vi "Bundle.vi"(6 "Combined Publish?":bool, 7 "Data Alias Array":string[](array[string]), 8 "error in (no error)":errorcluster, 9 "Message Array in":refnum<class "Message.lvclass">[](array[class]), 10 "Msg Alias":string, 11 "Reorder Driver Aliases Msg in":refnum<class "Custom Multi Instrument Msg.lvclass">) -> (0 "error out":errorcluster, 3 "Reorder Driver Aliases Msg out":refnum<class "Custom Multi Instrument Msg.lvclass">)   [LabVIEW 2020, in "Instrument Handler.lvlib" / "Custom Multi Instrument Msg.lvclass"]
doc: "Populate the Custom Multi Instrument Msg class."
uses:
  Custom Multi Instrument Msg.lvclass
  PPL/HDH.Actor Framework.Core.Actor.lvlibp/1abvi3w/vi.lib/ActorFramework/Message/Message.lvclass
  Custom Multi Instrument Msg.lvclass/Custom Multi Instrument Msg.ctl
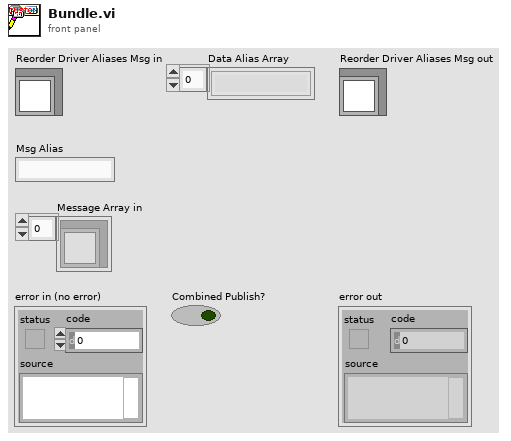
[diagram p1: front panel]
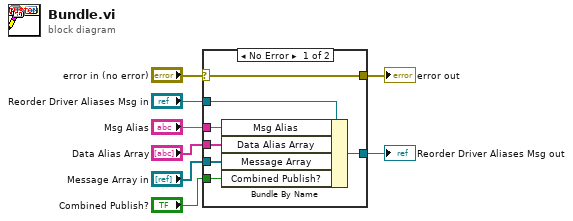
[diagram p0: block diagram]
diagram:
  n1 = case shown="No Error" "error in (no error)" {
    selector: "error in (no error)" -> [w15 w16]
    tunnel: [w15 w16] -> w7
    tunnel: [w13 w17] -> w5
    tunnel: "Reorder Driver Aliases Msg in" -> [w14 w17]
    tunnel: "Msg Alias" -> [w12 _]
    tunnel: "Data Alias Array" -> [w11 _]
    tunnel: "Message Array in" -> [w10 _]
    tunnel: "Combined Publish?" -> [w9 _]
    frame No Error {
      n2 = Bundle By Name(cluster=w14, "Msg Alias"=w12, "Data Alias Array"=w11, "Message Array"=w10, "Combined Publish?"=w9) -> (w13:refnum<class "Custom Multi Instrument Msg.lvclass">)
    }
    frame Error {
    }
  }
  "error out" <- w7
  "Reorder Driver Aliases Msg out" <- w5
